vi "Get Selected Controls - List of properties.vi"(8 "error in (no error)":errorcluster, 10 "List of Properties":string[](array[string]), 11 "Data in":T2) -> (0 "error out":errorcluster, 3 "Selected Ctrls - List of Properties":T1)   [LabVIEW 2020, in "Control Property Tree.lvlib"]
uses:
  Control Property Tree.lvlib
  Module Data--cluster.ctl
  Ctrl Properties Map Data.ctl
  Property array.ctl
  Selected Ctrls - List of Controls.ctl
  Selected Ctrls - List of Properties.ctl
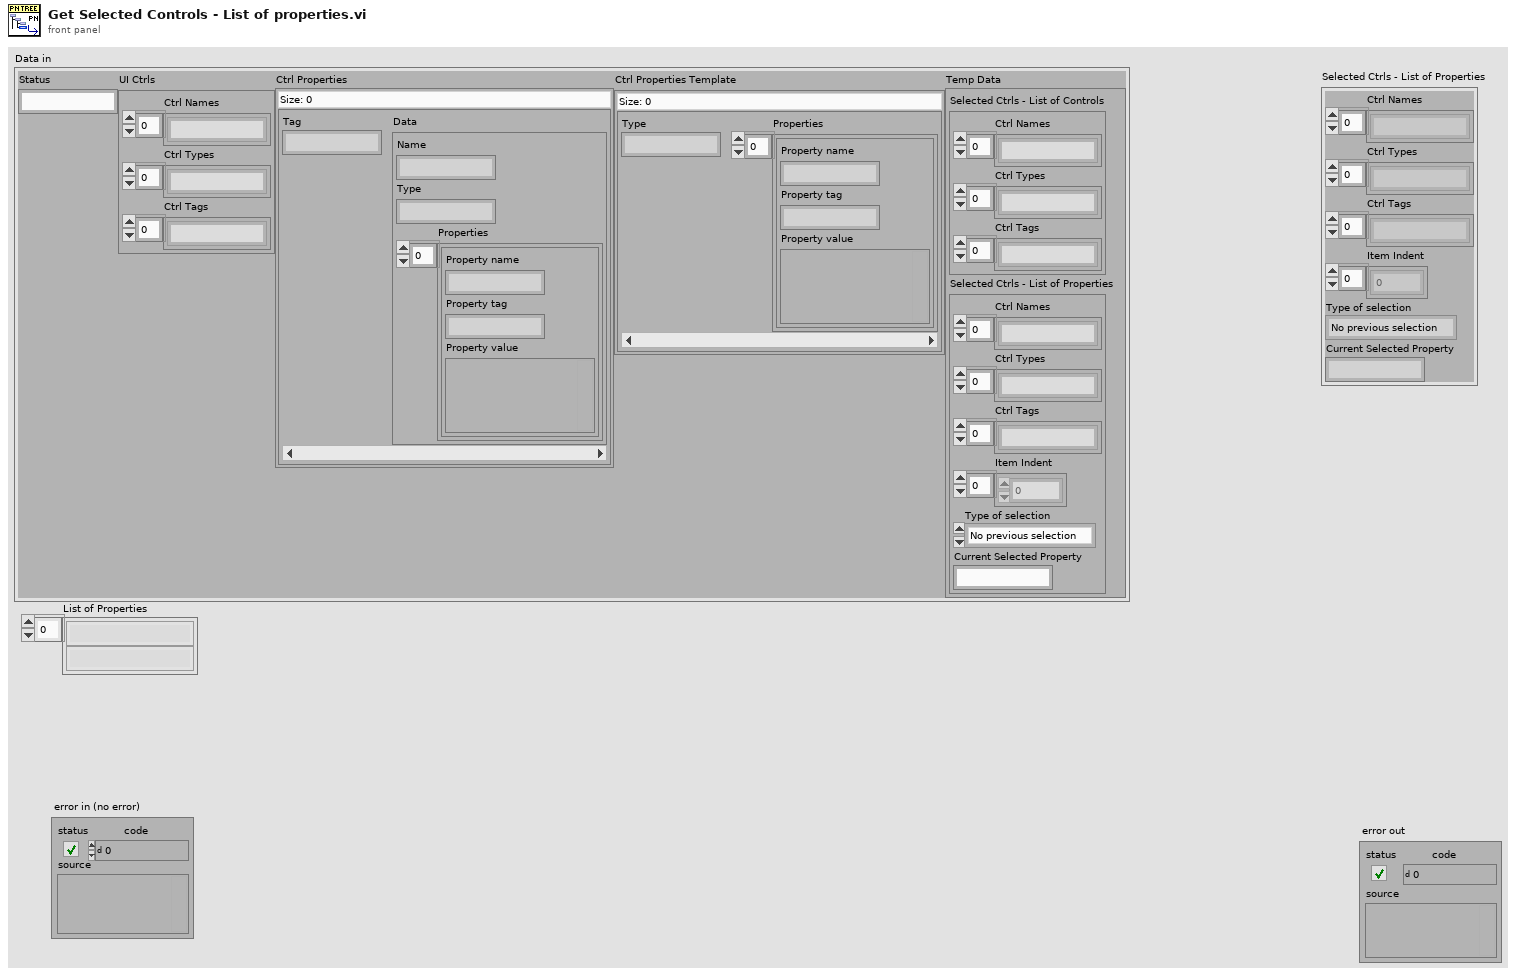
[diagram p1: front panel]
types:
  T1 = typedef "Control Property Tree.lvlib/Selected Ctrls - List of Properties.ctl" = cluster{"Ctrl Names":string[], "Ctrl Types":string[], "Ctrl Tags":string[], "Item Indent":i32[], "Type of selection":enum16{"No previous selection", "Control selected", "Property selected"}, "Current Selected Property":string}
  T2 = typedef "Control Property Tree.lvlib/Module Data--cluster.ctl" = cluster{"Status":string, "UI Ctrls":cluster{"Ctrl Names":string[], "Ctrl Types":string[], "Ctrl Tags":string[]}, "Ctrl Properties":map{string, T3}, "Ctrl Properties Template":map{string, T4}, "Temp Data":cluster{"Selected Ctrls - List of Controls":T5, "Selected Ctrls - List of Properties":T1}}
  T3 = typedef "Control Property Tree.lvlib/Ctrl Properties Map Data.ctl" = cluster{"Name":string, "Type":string, "Properties":T4}
  T4 = typedef "Control Property Tree.lvlib/Property array.ctl" = cluster{"Property name":string, "Property tag":string, "Property value":variant}[]
  T5 = typedef "Control Property Tree.lvlib/Selected Ctrls - List of Controls.ctl" = cluster{"Ctrl Names":string[], "Ctrl Types":string[], "Ctrl Tags":string[]}
  T6 = enum16{"No previous selection", "Control selected", "Property selected"}
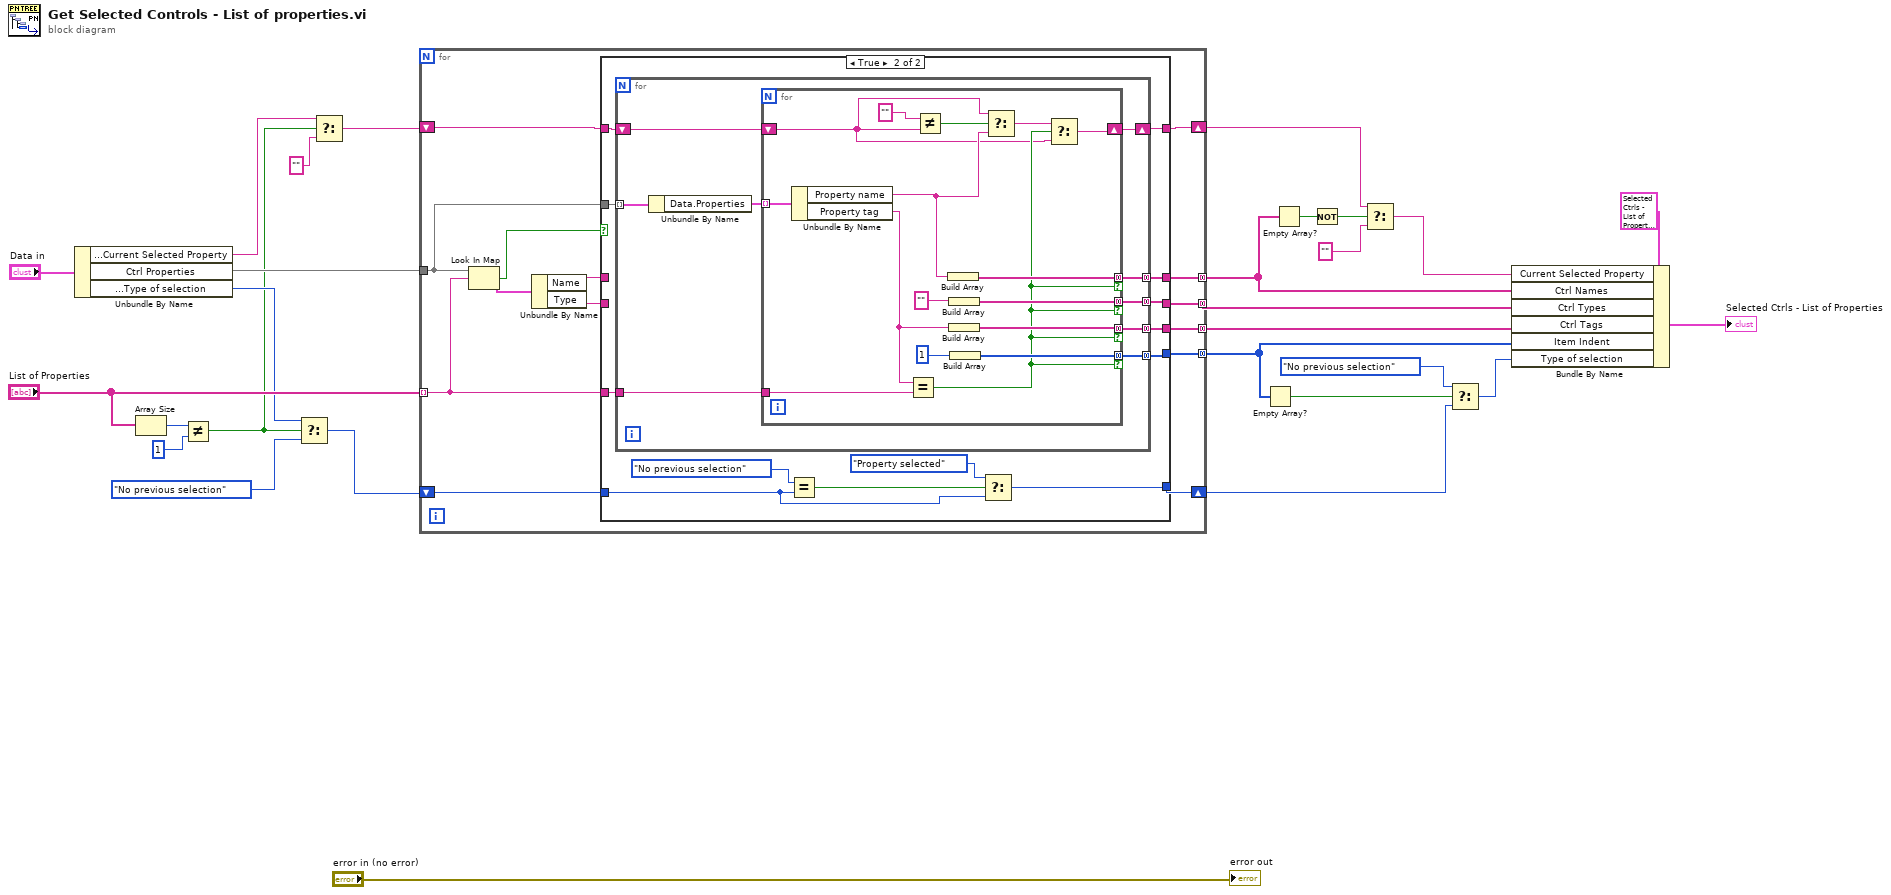
[diagram p0: block diagram]
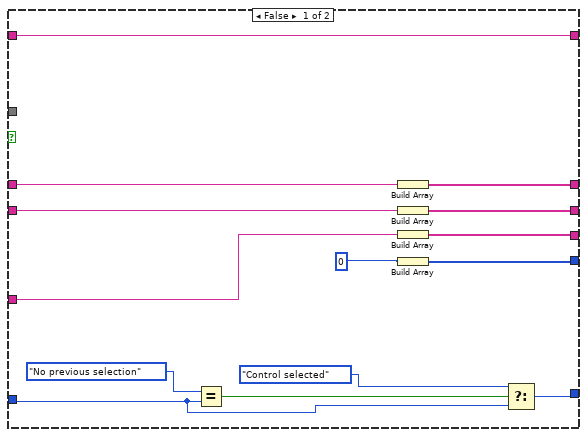
[diagram p2: hidden frame]
diagram:
  n1 = Unbundle By Name("Data in") -> ("Temp Data.Selected Ctrls - List of Properties.Current Selected Property"=w4:string, "Ctrl Properties"=w26:map{string, T3}, "Temp Data.Selected Ctrls - List of Properties.Type of selection"=w14:T6)
  n2 = Array Size(array="List of Properties") -> (size(s)=w16:i32)
  n3 = Not Equal?(x=w16, y=1) -> (x != y?=w1:bool)
  n4 = Select(t=w14, s=w1, f=T6."No previous selection") -> (s? t:f=w12:T6)
  n5 = Select(t=w4, s=w1, f="") -> (s? t:f=w3:string)
  n6 = for {
    tunnel: w26 -> [w41]
    tunnel: "List of Properties" -> [w38] mode=indexing
    tunnel: [w35] -> w10 mode=concatenating
    tunnel: [w37] -> w23 mode=concatenating
    tunnel: [w39] -> w22 mode=concatenating
    tunnel: [w33] -> w21 mode=concatenating
    shift-right: [w31] -> w19
    shift-left: w12 -> [w32]
    shift-right: [w29] -> w7
    shift-left: w3 -> [w30]
    n7 = Look In Map(map=w41, key=w38) -> (key not found?=w40:bool, value=w42:T3)  [unwired: 1 in]
    n8 = Unbundle By Name(w42) -> ("Name"=w34:string, "Type"=w36:string)
    n9 = case shown="True" w40 {
      tunnel: w41 -> [_ w69]
      tunnel: [w53 w66] -> w39
      tunnel: w38 -> [w52 w68]
      tunnel: [w55 w64] -> w37
      tunnel: w36 -> [w54 _]
      tunnel: [w56 w65] -> w35
      tunnel: w34 -> [w44 _]
      tunnel: [w50 w67] -> w33
      tunnel: w32 -> [w47 w62]
      tunnel: [w48 w61] -> w31
      tunnel: w30 -> [w43 w58]
      tunnel: [w43 w57] -> w29
      frame False {
        n10 = Equal?(x=T6."No previous selection" ("Temp Data.Selected Ctrls - List of Properties.Type of selection"), y=w47) -> (x = y?=w49:bool)
        n11 = Build Array(w44) -> (w56:string[])
        n12 = Build Array(w54) -> (w55:string[])
        n13 = Build Array(w52) -> (w53:string[])
        n14 = Build Array(0) -> (w50:i32[])
        n15 = Select(t=T6."Control selected" ("Temp Data.Selected Ctrls - List of Properties.Type of selection"), s=w49, f=w47) -> (s? t:f=w48:T6)
      }
      frame True {
        n16 = for {
          tunnel: w69 -> [w78] mode=indexing
          tunnel: w68 -> [w76]
          tunnel: [w75] -> w67 mode=concatenating
          tunnel: [w74] -> w66 mode=concatenating
          tunnel: [w73] -> w65 mode=concatenating
          tunnel: [w72] -> w64 mode=concatenating
          shift-right: [w70] -> w57
          shift-left: w58 -> [w71]
          n17 = Unbundle By Name(w78) -> ("Data.Properties"=w77:T4)
          n18 = for {
            tunnel: w77 -> [w94] mode=indexing
            tunnel: w76 -> [w93]
            tunnel: [w86] -> w75 mode=concatenating if=w81
            tunnel: [w91] -> w74 mode=concatenating if=w81
            tunnel: [w92] -> w73 mode=concatenating if=w81
            tunnel: [w88] -> w72 mode=concatenating if=w81
            shift-right: [w79] -> w70
            shift-left: w71 -> [w80]
            n19 = Unbundle By Name(w94) -> ("Property name"=w84:string, "Property tag"=w90:string)
            n20 = Equal?(x=w90, y=w93) -> (x = y?=w81:bool)
            n21 = Not Equal?(x="", y=w80) -> (x != y?=w83:bool)
            n22 = Build Array(w84) -> (w92:string[])
            n23 = Build Array("") -> (w88:string[])
            n24 = Build Array(w90) -> (w91:string[])
            n25 = Build Array(1) -> (w86:i32[])
            n26 = Select(t=w80, s=w83, f=w84) -> (s? t:f=w82:string)
            n27 = Select(t=w82, s=w81, f=w80) -> (s? t:f=w79:string)
          }
        }
        n28 = Equal?(x=T6."No previous selection" ("Temp Data.Selected Ctrls - List of Properties.Type of selection"), y=w62) -> (x = y?=w63:bool)
        n29 = Select(t=T6."Property selected" ("Temp Data.Selected Ctrls - List of Properties.Type of selection"), s=w63, f=w62) -> (s? t:f=w61:T6)
      }
    }
  }
  n30 = Empty Array?(array=w21) -> (empty?=w20:bool)
  n31 = Empty Array?(array=w10) -> (empty?=w9:bool)
  n32 = Not(x=w9) -> (.not. x?=w8:bool)
  n33 = Select(t=w7, s=w8, f="" ("x")) -> (s? t:f=w5:string)
  n34 = Select(t=T6."No previous selection" ("f"), s=w20, f=w19) -> (s? t:f=w18:T6)
  n35 = Bundle By Name(cluster=T1 {"Ctrl Names"=[], "Ctrl Types"=[], "Ctrl Tags"=[], "Item Indent"=[], "Type of selection"=enum."No previous selection", "Current Selected Property"=""} ("Selected Ctrls - List of Properties"), "Current Selected Property"=w5, "Ctrl Names"=w10, "Ctrl Types"=w23, "Ctrl Tags"=w22, "Item Indent"=w21, "Type of selection"=w18) -> (→"Selected Ctrls - List of Properties":T1)
  "error out" <- "error in (no error)"
